vi "macro_Translation2d_Dist_AngleDeg.vi"   [LabVIEW 2019, in "Trajectory_Library.lvlib"]
uses:
  Trajectory_Library.lvlib
types:
  T1 = typedef "Trajectory_Library.lvlib/ROTATION2D.ctl" = cluster{"VALUE":dbl, "COS":dbl, "SIN":dbl}
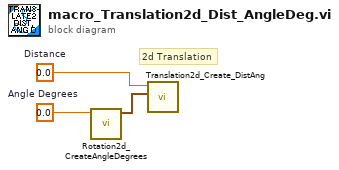
[diagram p0: block diagram]
diagram:
  w3 = 0.0  # Distance
  w1 = 0.0  # Angle Degrees
  # "2d Translation"
  n1 = call "Rotation2d_CreateAngleDegrees.vi"("Angle_Degrees"=w1) -> ("ROTATION"=w2:T1)  [unwired: 10 in]
  n2 = call "Translation2d_Create_DistAng.vi"("Angle"=w2, "Dist"=w3) -> ()  [unwired: 9 in, 1 out]
